vi "2.2 SailControlFunction.vi"(10 "Apparent Wind\nDirection":T4) -> (2 "Sail Position":T3, 9 "Which Boat Am I?":T2 items=["Small RC", "Large RC", "Final Boat", "Simulator"])   [LabVIEW 2011]
doc: "Sets the desired sail position based on the apparent wind direction.\nDesired sail position is same from 0-4 degrees, 5-9 degrees, and so on and so forth.\nValues come from a lookup table, which hopefully will make it easier to change if experimentation calls for different set values."
uses:
  2 Typedefs/apparent wind direction.ctl
  2 Typedefs/sail setpt.ctl
  2 Typedefs/Which Boat.ctl
  2 Globals/2 Global.vi
panel:
  out "Lookup Table":T1(tab)
  in  "Sail Setpoint Lookup Table Small RC - 72 elements, 0 - 360 degrees with changes only occurring at 5 degree increments":dbl[][](array[numeric])=[[0.0, 0.0, 0.0, 0.0, 0.0, 0.0, 0.0, 0.0, 0.0, 0.0, 0.055, 0.111, 0.166, 0.222, 0.277, 0.333, 0.388, 0.444, 0.5, 0.5278, 0.5556, 0.5833, 0.6111, 0.6389, 0.6667, 0.6944, 0.7222, 0.75, 0.7778, 0.8056, 0.8333, 0.8611, 0.8889, 0.9167, 0.9444, 0.9722, 1.0], [1.0, 0.9722, 0.9444, 0.9167, 0.8889, 0.8611, 0.8333, 0.8056, 0.7778, 0.75, 0.7222, 0.6944, 0.6667, 0.6389, 0.6111, 0.5833, 0.5556, 0.5278, 0.5, 0.4444, 0.3889, 0.3333, 0.2778, 0.2222, 0.1667, 0.1111, 0.0556, 0.0, 0.0, 0.0, 0.0, 0.0, 0.0, 0.0, 0.0, 0.0, 0.0]]
  in  "Sail Setpoint Lookup Table Large RC - 72 elements, 0 - 360 degrees with changes only occurring at 5 degree increments":dbl[][](array[numeric])=[[0.0, 0.0, 0.0, 0.0, 0.0, 0.0, 0.0, 0.0, 0.0, 0.0, 0.055, 0.111, 0.166, 0.222, 0.277, 0.333, 0.388, 0.444, 0.5, 0.5278, 0.5556, 0.5833, 0.6111, 0.6389, 0.6667, 0.6944, 0.7222, 0.75, 0.7778, 0.8056, 0.8333, 0.8611, 0.8889, 0.9167, 0.9444, 0.9722, 1.0], [1.0, 0.9722, 0.9444, 0.9167, 0.8889, 0.8611, 0.8333, 0.8056, 0.7778, 0.75, 0.7222, 0.6944, 0.6667, 0.6389, 0.6111, 0.5833, 0.5556, 0.5278, 0.5, 0.4444, 0.3889, 0.3333, 0.2778, 0.2222, 0.1667, 0.1111, 0.0556, 0.0, 0.0, 0.0, 0.0, 0.0, 0.0, 0.0, 0.0, 0.0, 0.0]]
  in  "Sail Setpoint Lookup Table Final Boat - 72 elements, 0 - 360 degrees with changes only occurring at 5 degree increments":dbl[][](array[numeric])=[[0.0, 0.0, 0.0, 0.0, 0.0, 0.0, 0.0, 0.0, 0.0, 0.0, 0.055, 0.111, 0.166, 0.222, 0.277, 0.333, 0.388, 0.444, 0.5, 0.5278, 0.5556, 0.5833, 0.6111, 0.6389, 0.6667, 0.6944, 0.7222, 0.75, 0.7778, 0.8056, 0.8333, 0.8611, 0.8889, 0.9167, 0.9444, 0.9722, 1.0], [1.0, 0.9722, 0.9444, 0.9167, 0.8889, 0.8611, 0.8333, 0.8056, 0.7778, 0.75, 0.7222, 0.6944, 0.6667, 0.6389, 0.6111, 0.5833, 0.5556, 0.5278, 0.5, 0.4444, 0.3889, 0.3333, 0.2778, 0.2222, 0.1667, 0.1111, 0.0556, 0.0, 0.0, 0.0, 0.0, 0.0, 0.0, 0.0, 0.0, 0.0, 0.0]]
  in  "Sail Setpoint Lookup Table Simulator- 72 elements, 0 - 360 degrees with changes only occurring at 5 degree increments":dbl[][](array[numeric])=[[0.0, 0.0, 0.0, 0.0, 0.0, 0.0, 0.0, 0.0, 0.0, 0.0, 0.055, 0.111, 0.166, 0.222, 0.277, 0.333, 0.388, 0.444, 0.5, 0.5278, 0.5556, 0.5833, 0.6111, 0.6389, 0.6667, 0.6944, 0.7222, 0.75, 0.7778, 0.8056, 0.8333, 0.8611, 0.8889, 0.9167, 0.9444, 0.9722, 1.0], [1.0, 0.9722, 0.9444, 0.9167, 0.8889, 0.8611, 0.8333, 0.8056, 0.7778, 0.75, 0.7222, 0.6944, 0.6667, 0.6389, 0.6111, 0.5833, 0.5556, 0.5278, 0.5, 0.4444, 0.3889, 0.3333, 0.2778, 0.2222, 0.1667, 0.1111, 0.0556, 0.0, 0.0, 0.0, 0.0, 0.0, 0.0, 0.0, 0.0, 0.0, 0.0]]
  # "First row is 0-180\nSecond row is 180-360, and in theory should be equal to the first one. Experiments must be run to determine if this is true."
  # "Currently 0 from 0-45, straight line 50 - 90 (.5), straight line 95 - 180 (1)"
  # "90"
  # "180"
  # "135"
  # "270"
  # "225"
  # "315"
  # "360"
  # "90"
  # "135"
  # "180"
  # "270"
  # "360"
  # "225"
  # "315"
  # "90"
  # "135"
  # "180"
  # "225"
  # "270"
  # "315"
  # "360"
  # "90"
  # "135"
  # "180"
  # "315"
  # "360"
  # "225"
  # "270"
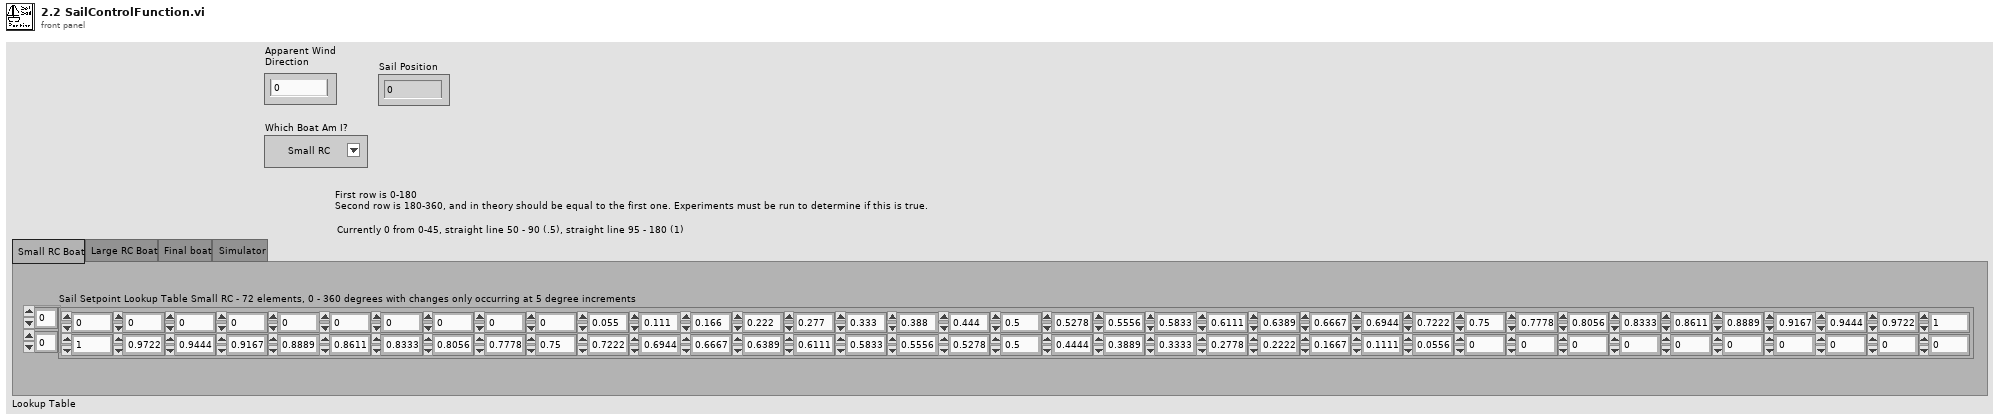
[diagram p1: front panel]
types:
  T1 = enum32{"Small RC Boat", "Large RC Boat", "Final boat", "Simulator "}
  T2 = typedef "Which Boat.ctl" = u16
  T3 = typedef "sail setpt.ctl" = dbl
  T4 = typedef "apparent wind direction.ctl" = dbl
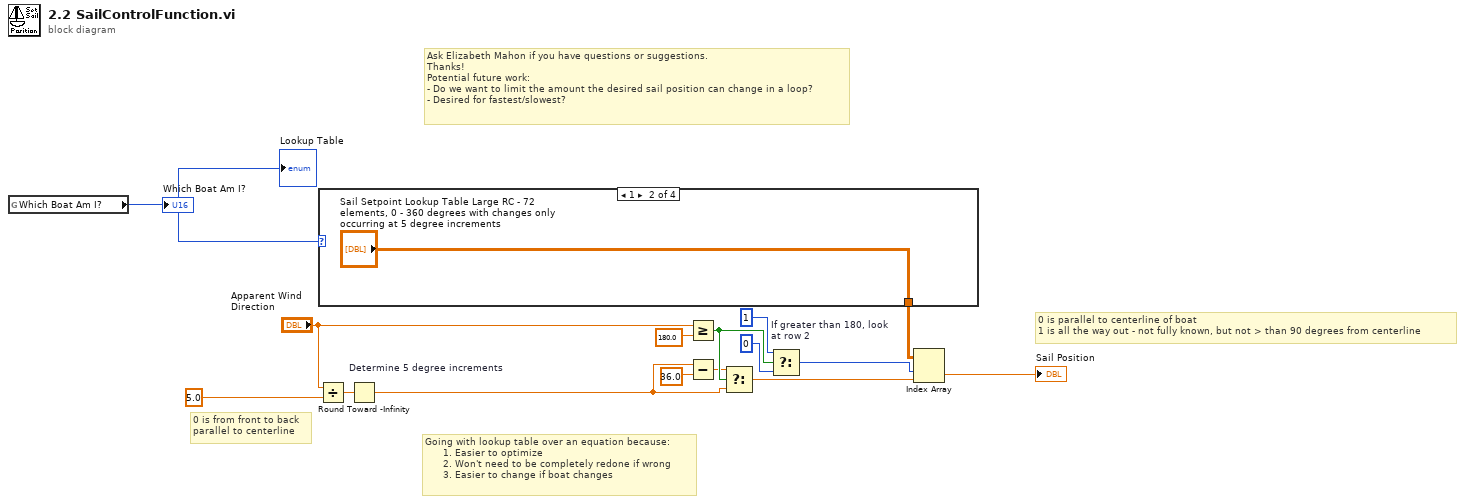
[diagram p0: block diagram]
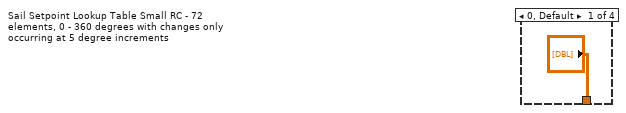
[diagram p2: hidden frame]
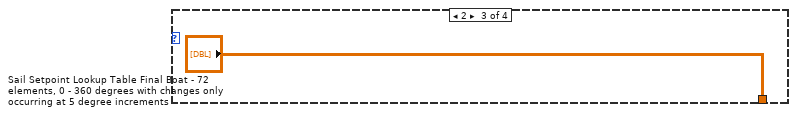
[diagram p3: hidden frame]
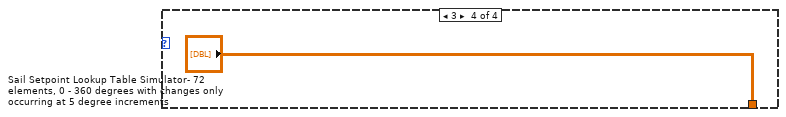
[diagram p4: hidden frame]
diagram:
  # "0 is from front to back\nparallel to centerline"
  # "Ask Elizabeth Mahon if you have questions or suggestions.\nThanks!\nPotential future work:\n- Do we want to limit the amount the desired sail position can change in a loop?\n- Desired for fastest/slowest?"
  # "0 is parallel to centerline of boat\n1 is all the way out - not fully known, but not > than 90 degrees from centerline"
  # "Going with lookup table over an equation because:\n      1. Easier to optimize\n      2. Won't need to be completely redone if wrong\n      3. Easier to change if boat changes"
  n1 = global read "2 Global.vi" "Which Boat Am I?"() -> (w1:T2)
  "Which Boat Am I?" <- w1
  "Lookup Table" <- w1
  n2 = Divide(x="Apparent Wind\nDirection", y=T4 5.0) -> (x/y=w13:T4)
  n3 = case shown="1" w1 {
    tunnel: ["Sail Setpoint Lookup Table Small RC - 72 elements, 0 - 360 degrees with changes only occurring at 5 degree increments" "Sail Setpoint Lookup Table Large RC - 72 elements, 0 - 360 degrees with changes only occurring at 5 degree increments" "Sail Setpoint Lookup Table Final Boat - 72 elements, 0 - 360 degrees with changes only occurring at 5 degree increments" "Sail Setpoint Lookup Table Simulator- 72 elements, 0 - 360 degrees with changes only occurring at 5 degree increments"] -> w7
    frame 0, Default {
    }
    frame 1 {
    }
    frame 2 {
    }
    frame 3 {
    }
  }
  n4 = Round Toward -Infinity "Determine 5 degree increments"(1:w13) -> (0:w3:T4)
  n5 = Greater Or Equal?(x="Apparent Wind\nDirection", y=T4 180.0) -> (x >= y?=w6:bool)
  n6 = Subtract(x=w3, y=T4 36.0) -> (x-y=w4:T4)
  n7 = Select(t=w4, s=w6, f=w3) -> (s? t:f=w2:T4)
  n8 = Select "If greater than 180, look\nat row 2"(t=1, s=w6, f=0) -> (s? t:f=w8:i32)
  n9 = Index Array(array=w7, index (row)=w8, index (col)=w2) -> (element=→"Sail Position":dbl)
